vi "QTMDriver.vi"(0 "connection ID":refnum<k5>, 1 "DataIn":dbl[](array[numeric]), 2 "DataOutIndex":i32, 3 "error in":errorcluster, 4 "Ring":T1) -> (7 "connection ID out":refnum<k5>, 8 "DataOut":dbl[](array[numeric]), 10 "error out":errorcluster)   [LabVIEW 2010]
uses:
  CustomIO.ctl
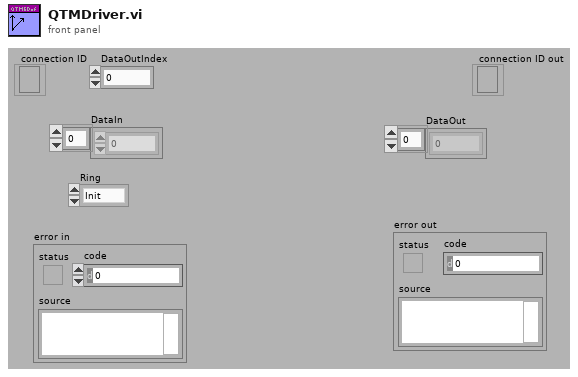
[diagram p1: front panel]
types:
  T1 = typedef "CustomIO.ctl" = enum16{"Init", "Read", "Write", "Close", "N/O"}
  T2 = typedef "QTM Data Frame.ctl" = cluster{"Timestamp":i64, "Framenumber":i32, "ComponentCount":i32, "Components":cluster{"ComponentSize":i32, "ComponentType":T3, "Count":i32, "Padding":i32, "Data":dbl[][]}[]}
  T3 = typedef "QTM ComonentType.ctl" = i32
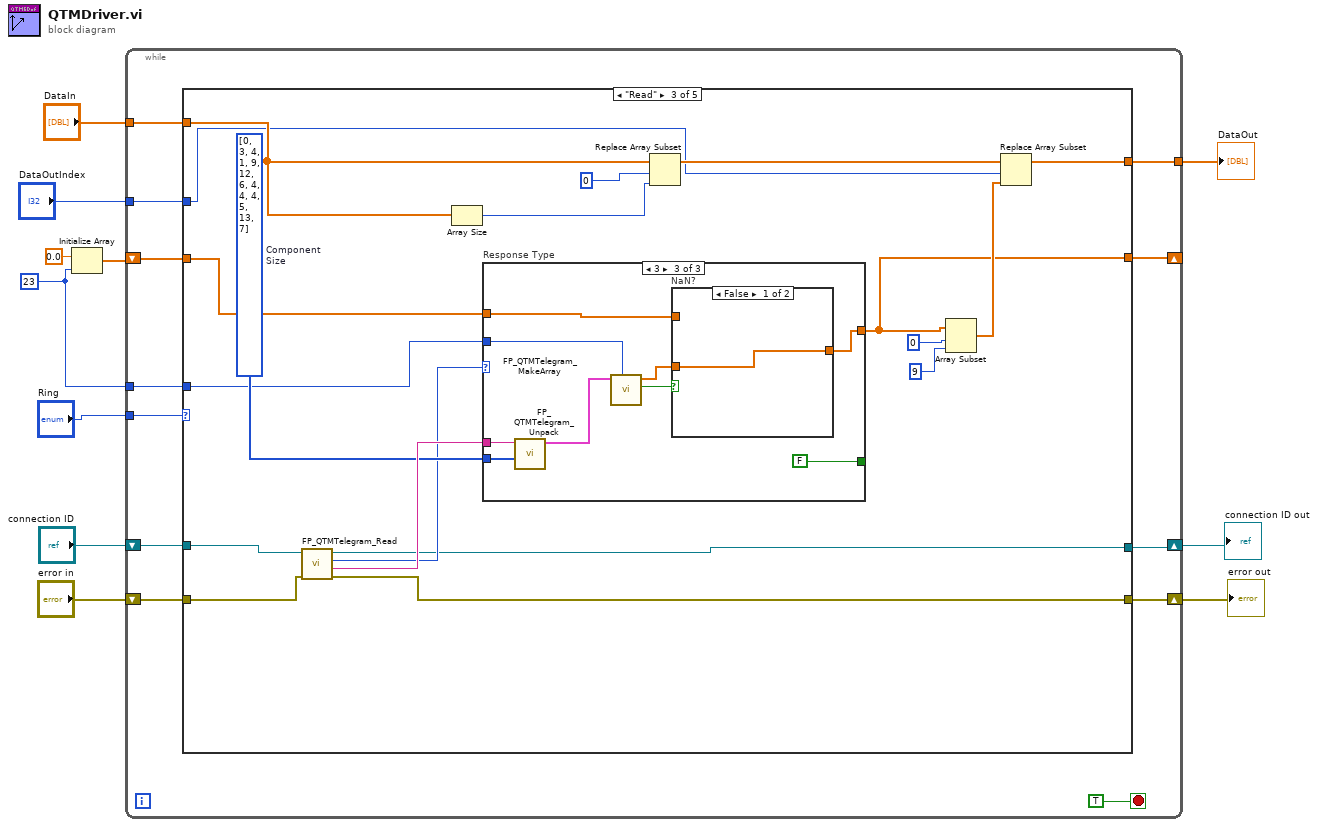
[diagram p0: block diagram]
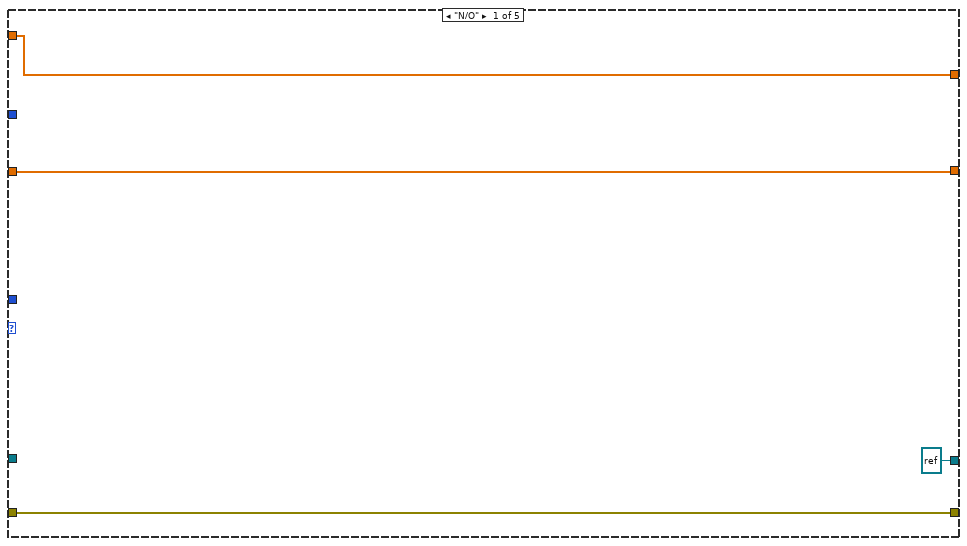
[diagram p2: hidden frame]
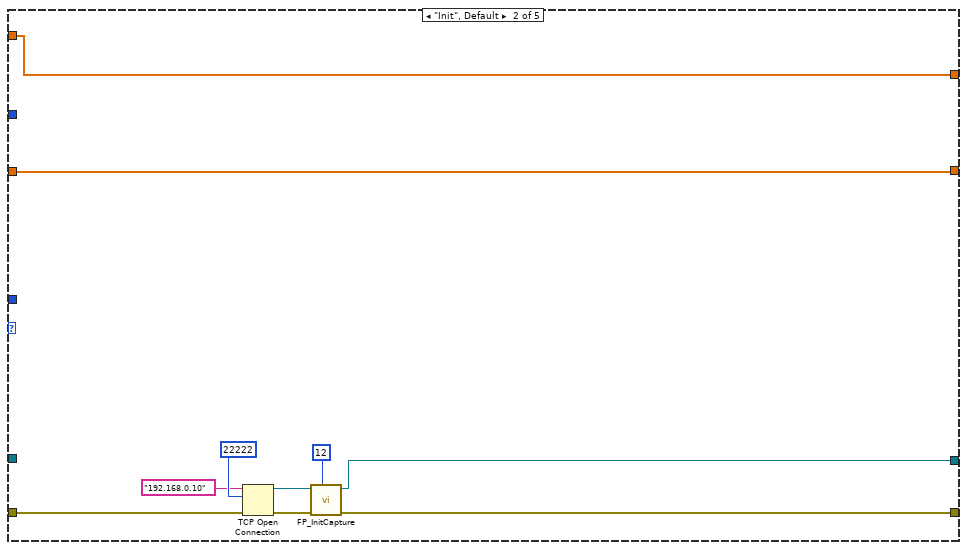
[diagram p3: hidden frame]
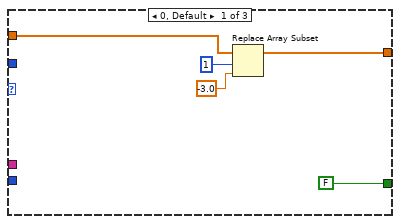
[diagram p4: hidden frame]
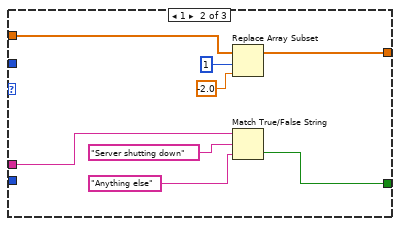
[diagram p5: hidden frame]
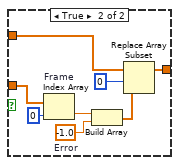
[diagram p6: hidden frame]
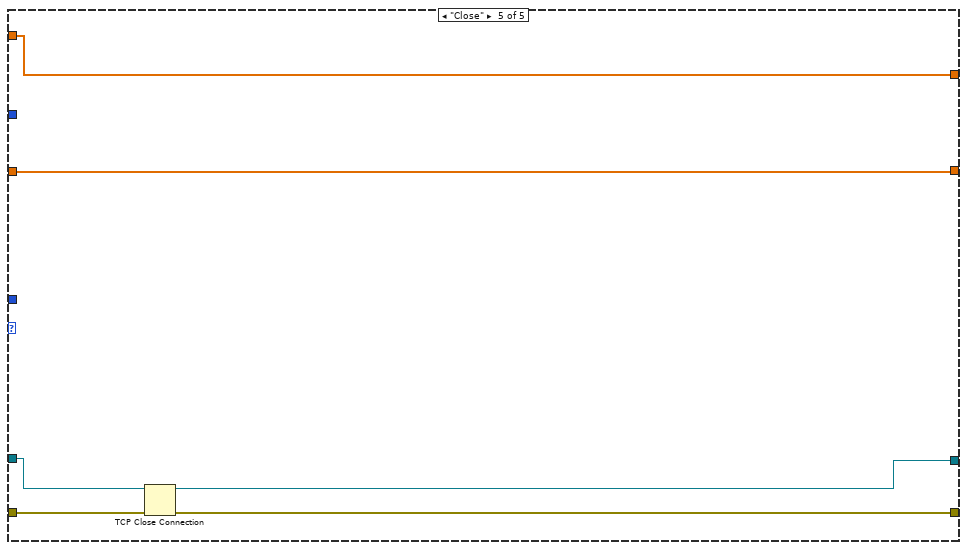
[diagram p8: hidden frame]
diagram:
  w8 = 23
  n1 = Initialize Array(0.0 ("element"), w8) -> (w9:dbl[])
  n2 = while {
    tunnel: "Ring" -> [w23]
    shift-right: [w21] -> _
    shift-left: w9 -> [w20]
    tunnel: w8 -> [w19]
    shift-right: [w17] -> w6
    shift-left: "error in" -> [w18]
    shift-right: [w15] -> w4
    shift-left: "connection ID" -> [w16]
    tunnel: "DataIn" -> [w14]
    tunnel: [w13] -> w2
    tunnel: "DataOutIndex" -> [w12]
    stop <- TRUE stop-if-true
    n3 = case shown="\"Read\"" w23 {
      tunnel: [w27 w30 w46 w91 w93] -> w21
      tunnel: w20 -> [w27 w30 w47 w91 w93]
      tunnel: w19 -> [_ _ w45 _ _]
      tunnel: w18 -> [w26 w31 w44 w89 w96]
      tunnel: [w26 w32 w43 w89 w95] -> w17
      tunnel: w16 -> [_ _ w42 w90 w97]
      tunnel: [refnum<k5> refnum ("connection ID") w33 w41 w90 w94] -> w15
      tunnel: w14 -> [w24 w29 w40 w88 w92]
      tunnel: [w24 w29 w39 w88 w92] -> w13
      tunnel: w12 -> [_ _ w38 _ _]
      frame "N/O" {
      }
      frame "Init", Default {
        n4 = TCP Open Connection(address="192.168.0.10", remote port or service name=u16 22222, error in (no error)=w31) -> (connection ID=w37:refnum<k5>, error out=w36:errorcluster)  [unwired: 2 in]
        n5 = call "FP_InitCapture.vi"("ComponentType"=u32 12, "error out 2"=w36, "connection ID"=w37) -> ("error out"=w32:errorcluster, "connection ID out"=w33:refnum<k5>)  [unwired: 5 in, 2 out]
      }
      frame "Read" {
        w55 = i32[] [0, 3, 4, 1, 9, 12, 6, 4, 4, 4, 5, 13, 7]  # Component Size
        n6 = call "FP_QTMTelegram_Read.vi"("error in (no error)"=w44, "connection ID in"=w42) -> ("error out"=w43:errorcluster, "Data"=w56:string, "Response type"=w50:i32, "connection ID out"=w41:refnum<k5>)  [unwired: 6 out]
        n7 = Array Size(array=w40) -> (size(s)=w49:i32)
        n8 = case "Response Type" shown="3" w50 {
          tunnel: w56 -> [_ w67 w77]
          tunnel: [FALSE ("selection") w66 FALSE ("selection")] -> _
          tunnel: [w59 w63 w74] -> w46
          tunnel: w55 -> [_ _ w72]
          tunnel: w45 -> [_ _ w71]
          tunnel: w47 -> [w57 w62 w70]
          frame 0, Default {
            n9 = Replace Array Subset(array=w57, new element=sgl -3.0 ("new element/subarray"), index=1) -> (w59:dbl[])
          }
          frame 1 {
            n10 = Replace Array Subset(array=w62, new element=sgl -2.0 ("new element/subarray"), index=1) -> (w63:dbl[])
            n11 = Match True/False String(2:"Anything else" ("false string"), 3:"Server shutting down" ("true string"), 4:w67) -> (0:w66:bool)  [unwired: 1 out]
          }
          frame 3 {
            n12 = call "FP_QTMTelegram_Unpack.vi"("Component\nSize"=w72, "6DOF telegram"=w77) -> ("Data Frame"=w73:T2)  [unwired: 9 out]
            n13 = call "FP_QTMTelegram_MakeArray.vi"("Array\nSize"=w71, "Data Frame"=w73) -> ("NaN?"=w76:bool, "ArrayOut"=w75:dbl[])  [unwired: 8 out]
            n14 = case "NaN?" shown="False" w76 {
              tunnel: w75 -> [w79 w85]
              tunnel: [w79 w86] -> w74
              tunnel: w70 -> [_ w80]
              frame False {
              }
              frame True {
                w82 = sgl -1.0  # Error
                n15 = Index Array "Frame"(array=w85, index=0) -> (element=w83:dbl)
                n16 = Build Array(w83, w82) -> (w81:dbl[])
                n17 = Replace Array Subset(array=w80, new element=w81, index=0) -> (w86:dbl[])
              }
            }
          }
        }
        n18 = Replace Array Subset(array=w40, new element=w49, index=0) -> (w51:dbl[])
        n19 = Array Subset(array=w46, index=0, length=9) -> (w48:dbl[])
        n20 = Replace Array Subset(array=w51, new element=w48, index=w38) -> (w39:dbl[])
      }
      frame "Write" {
      }
      frame "Close" {
        n21 = TCP Close Connection(connection ID=w97, error in (no error)=w96) -> (connection ID out=w94:refnum<k5>, error out=w95:errorcluster)  [unwired: 1 in]
      }
    }
  }
  "error out" <- w6
  "connection ID out" <- w4
  "DataOut" <- w2
